vi "FindSignalTransform.vi"(2 "Desired data":string="microphone", 3 "Data Sets In":T1[](array[typedef]) {"Settings"."Time" format="%<%H:%M\n%d/%m/%y>T"}) -> (0 "Coherence":cluster{dbl, "df":dbl, dbl[]}[](graph), 1 "Spectra Out":T1[](array[typedef]) {"Settings"."Time" format="%<%H:%M\n%d/%m/%y>T"})   [LabVIEW 2014]
uses:
  <userlib>/CurtinCode/DataControl.ctl
  <userlib>/CurtinCode/SettingsControl.ctl
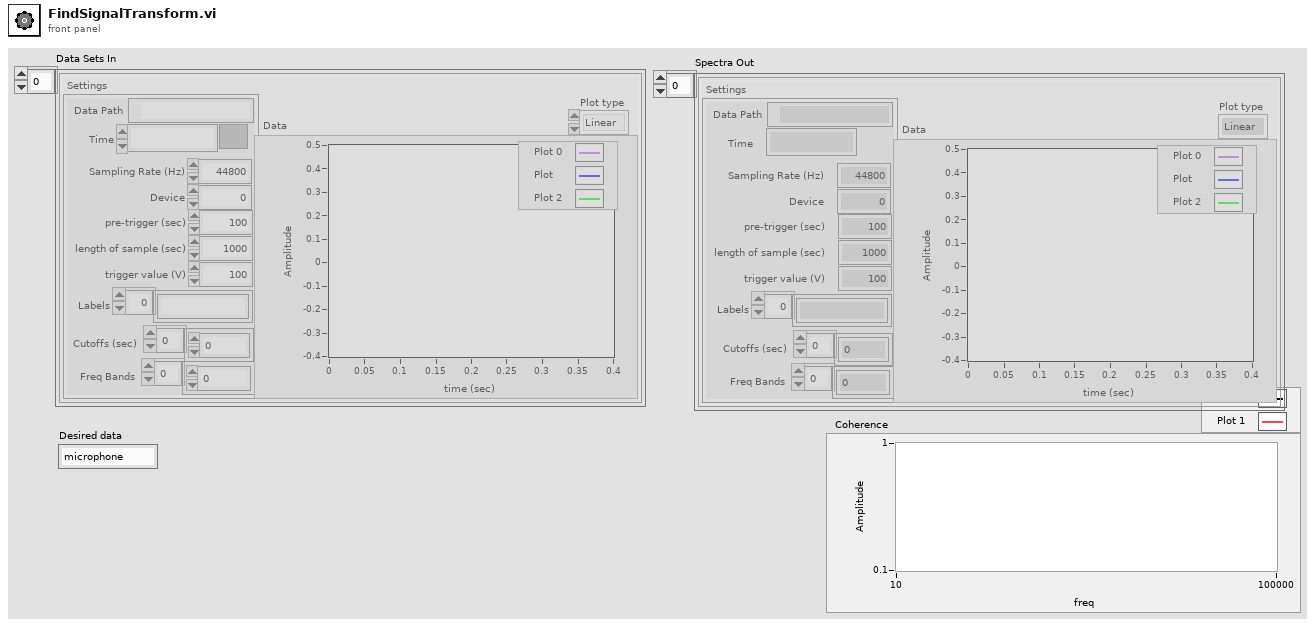
[diagram p1: front panel]
types:
  T1 = typedef "DataControl.ctl" = cluster{"Settings":T2, "Data":cluster{i32, dbl, "data":dbl[]}[], "Plot type":enum16{"Linear", "log"}}
  T2 = typedef "SettingsControl.ctl" = cluster{"Data Path":path, "Time":timestamp, "Sampling Rate (Hz)":u16, "Device":u16, "pre-trigger (sec)":dbl, "length of sample (sec)":dbl, "trigger value (V)":dbl, "Labels":string[], "Cutoffs (sec)":dbl[], "Freq Bands":dbl[]}
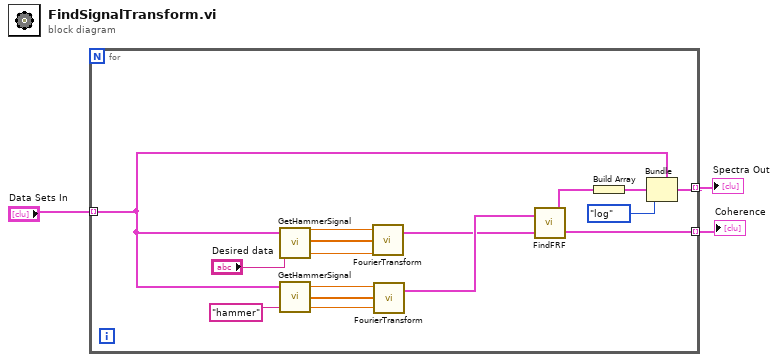
[diagram p0: block diagram]
diagram:
  n1 = for {
    tunnel: [w6] -> w3 mode=indexing
    tunnel: "Data Sets In" -> [w11] mode=indexing
    tunnel: [w9] -> w1 mode=indexing
    n2 = call <userlib>:"GetHammerSignal.vi"("column"="Desired data", "Data Set"=w11) -> ("Cutoff"=w13:dbl, "Data set"=w16:dbl[], "time between samples"=w17:dbl)  [unwired: 1 in]
    n3 = call <userlib>:"GetHammerSignal.vi"("column"="hammer", "Data Set"=w11) -> ("Cutoff"=w12:dbl, "Data set"=w14:dbl[], "time between samples"=w15:dbl)  [unwired: 1 in]
    n4 = call <userlib>:"FourierTransform.vi"("Cutoff (s)"=w13, "Time Data"=w16, "time per sample"=w17) -> ("FFT"=w4:cluster{dbl, "df":dbl, "FFT {X}":cdb[]})  [unwired: 1 out]
    n5 = call <userlib>:"FourierTransform.vi"("Cutoff (s)"=w12, "Time Data"=w14, "time per sample"=w15) -> ("FFT"=w5:cluster{dbl, "df":dbl, "FFT {X}":cdb[]})  [unwired: 1 out]
    n6 = call <userlib>:"FindFRF.vi"("Microphone FFT"=w4, "Hammer FFT"=w5) -> ("Coherence"=w6:cluster{dbl, "df":dbl, dbl[]}, "Current FRF"=w7:cluster{dbl, "df":dbl, dbl[]})
    n7 = Build Array(w7) -> (w10:cluster{dbl, "df":dbl, dbl[]}[])
    n8 = Bundle(cluster=w11, "Data"=w10, "Plot type"=enum16{"Linear", "log"}."log") -> (w9:T1)  [unwired: 1 in]
  }
  "Coherence" <- w3
  "Spectra Out" <- w1
